vi "mxwScript_API_XMLChainConnections.vi"(5 "internal?":bool, 6 "connect last":T1={"connect?"=FALSE, "final label"="", "use index?"=FALSE, "connPaneIndex"=0, "area"=enum."TopLeft", "connection type"=enum."Recommended"}, 7 "connect first":T1={"connect?"=FALSE, "final label"="", "use index?"=FALSE, "connPaneIndex"=0, "area"=enum."TopLeft", "connection type"=enum."Recommended"}, 8 "error in (no error)":errorcluster, 9 "diagram ID":string="mxwRoot", 10 "sink pattern":string, 11 "source pattern":string) -> (0 "error out":errorcluster, 3 "template connection":T4)   [LabVIEW 2020]
uses:
  codeGenAPISupport.llb/cgAPI_mxwScript_Wire_InputWireConnection.ctl
  codeGenAPISupport.llb/cgAPI_mxwScript_Wire_ChnCnnctStartEndData.ctl
  codeGenAPISupport.llb/cgAPI_mxwScript_ConnPaneArea.ctl
  codeGenAPISupport.llb/cgAPI_mxwScript_ConnPaneConnectionType.ctl
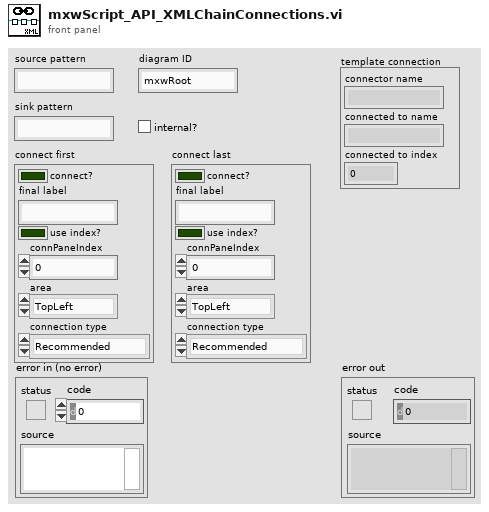
[diagram p1: front panel]
types:
  T1 = typedef "cgAPI_mxwScript_Wire_ChnCnnctStartEndData.ctl" = cluster{"connect?":bool, "final label":string, "use index?":bool, "connPaneIndex":i32, "area":T2, "connection type":T3}
  T2 = typedef "cgAPI_mxwScript_ConnPaneArea.ctl" = enum16{"TopLeft", "Top", "TopRight", "Right", "BottomRight", "Bottom", "BottomLeft", "Left"}
  T3 = typedef "cgAPI_mxwScript_ConnPaneConnectionType.ctl" = enum16{"Invalid Wire Rule", "Required", "Recommended", "Optional", "Dynamic Dispatch"}
  T4 = typedef "cgAPI_mxwScript_Wire_InputWireConnection.ctl" = cluster{"connector name":string, "connected to name":string, "connected to index":i32}
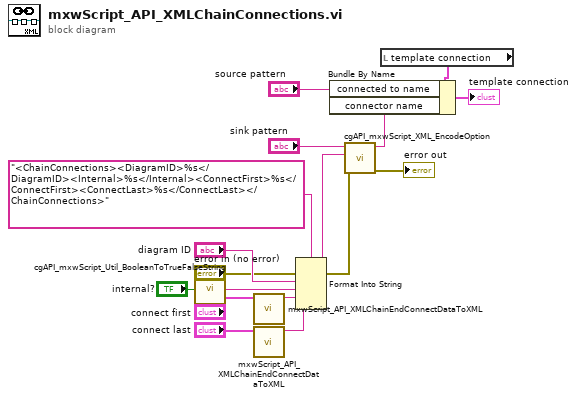
[diagram p0: block diagram]
diagram:
  n1 = call "cgAPI_mxwScript_Util_BooleanToTrueFalseString.vi"("boolean"="internal?") -> ("TRUE/FALSE text"=w1:string)  [unwired: 4 out]
  n2 = call "mxwScript_API_XMLChainEndConnectDataToXML.vi"("connect in"="connect first") -> ("ConnectXML"=w9:string)  [unwired: 1 in, 9 out]
  n3 = call "mxwScript_API_XMLChainEndConnectDataToXML.vi"("connect in"="connect last") -> ("ConnectXML"=w8:string)  [unwired: 1 in, 9 out]
  n4 = Format Into String(format string="<ChainConnections><DiagramID>%s</DiagramID><Internal>%s</Internal><ConnectFirst>%s</ConnectFirst><ConnectLast>%s</ConnectLast></ChainConnections>", error in="error in (no error)", "diagram ID", w1, w9, w8) -> (resulting string=w7:string, error out=w5:errorcluster)  [unwired: 1 in]
  n5 = call "cgAPI_mxwScript_XML_EncodeOption.vi"("error in (no error)"=w5, "otherXML"=w7, "normalTextString"="sink pattern") -> ("error out"=→"error out":errorcluster, "encodedString"=w3:string)  [unwired: 7 out]
  n6 = local read "template connection"() -> (w15:T4)
  n7 = Bundle By Name(cluster=w15, "connected to name"="source pattern", "connector name"=w3) -> (→"template connection":T4)
